vi "Compute Colour Pair.vi"(5 "Fractional Scale Upper":sgl=0.1, 7 "Fractional Scale Lower":sgl=0.1, 8 "error in (no error)":errorcluster, 11 "Starting Colour":u32(colorbox)) -> (0 "error out":errorcluster, 3 "Colour Pair":T1)   [LabVIEW 2020, in "g_ar_toolkit.image.lvlib"]
uses:
  g_ar_toolkit.image.lvlib
  In-Range Image Colour Range.ctl
  g_ar_toolkit.common/g_ar_toolkit.common.lvlib
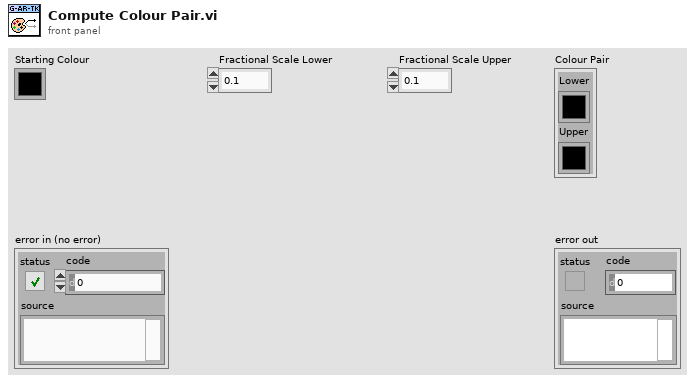
[diagram p1: front panel]
types:
  T1 = typedef "g_ar_toolkit.image.lvlib/In-Range Image Colour Range.ctl" = cluster{"Lower":u32, "Upper":u32}
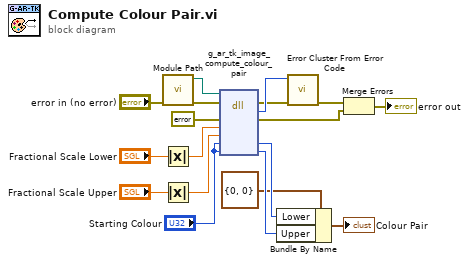
[diagram p0: block diagram]
diagram:
  n1 = call "Module Path.vi"("error in (no error)"="error in (no error)") -> ("error out"=w15:errorcluster, "Path"=w18:path)  [unwired: 9 in]
  n2 = Absolute Value(x="Fractional Scale Lower") -> (abs(x)=w13:sgl)
  n3 = Absolute Value(x="Fractional Scale Upper") -> (abs(x)=w1:sgl)
  n4 = dll-call lib="?" fn="g_ar_tk_image_compute_colour_pair" ("g_ar_toolkit.*.*:g_ar_tk_image_get_text_size")(path in=w18, error in=w15, "error"=errorcluster {"status"=FALSE, "code"=0, "source"=""} ("error constant"), "Fractional_Scale_Lower"=w13, "Fractional_Scale_Upper"=w1, "Darker"="Starting Colour", "Lighter"="Starting Colour") -> (error out=w16:errorcluster, "MgErr"=w17:i32, "error"=w5:errorcluster, "Darker"=w12:u32, "Lighter"=w11:u32)  [unwired: 3 in, 1 out]
  n5 = Bundle By Name(cluster=T1 {"Lower"=0, "Upper"=0} ("In-Range Image Colour Range"), "Lower"=w12, "Upper"=w11) -> (→"Colour Pair":T1)
  n6 = call <vilib>:"Error Cluster From Error Code.vi"("error in (no error)"=w16, "error code (0)"=w17) -> ("error out"=w9:errorcluster)  [unwired: 7 in]
  n7 = Merge Errors(w9, w5) -> (→"error out":errorcluster)
